vi "Pfeiffer-RVC300.get revision.vi"(0 "i ref in":refnum<vi>, 3 "ms timeout (10000)":i32=10000, 5 "error in (no error)":errorcluster) -> (14 "i ref out":refnum<vi>, 16 "revision":string, 17 "timed out":bool, 19 "error out":errorcluster)   [LabVIEW 2014, in "Pfeiffer-RVC300.lvlib"]
doc: "Queries the revision number from the device and creates the deviceID.\n\nLicense Agreement for this software:\n\nCopyright (C)\nMax-Planck-Institut für Kernphysik\nSaupfercheckweg 1\n69117 Heidelberg\nGermany\n\nContact: christopher.borgmann@mpi-hd.mpg.de\n\nThis program is free software: you can redistribute it and/or modify \nit under the terms of the GNU General Public License as published by\nthe Free Software Foundation, either version 3 of the License, or\n(at your option) any later version.\n\nThis program is distributed in the hope that it will be useful,\nbut WITHOUT ANY WARRANTY; without even the implied warranty of\nMERCHANTABILITY or FITNESS FOR A PARTICULAR PURPOSE. See the\nGNU General Public License for more details.\n\nYou should have received a copy of the GNU General Public License\nalong with this program. If not, see <http://www.gnu.org/licenses/>.\n\nMax-Planck-Institut für Kernphysik\nSaupfercheckweg 1, 69117 Heidelberg, Germany\nFor all questions and ideas contact: christopher.borgmann@mpi-hd.mpg.de\nLast update: 08.07.2010"
uses:
  Pfeiffer-RVC300.lvlib
  CSCore/CSApplicationBaseClasses/DeviceBase/DeviceBase.lvlib
  CSlibraries-extern/DimLVEvent/NodeMon-LV/LVNodeInfo/LVNodeInfo.lvlib
  CSlibraries/UtilityLib/UtilityLib.lvlib
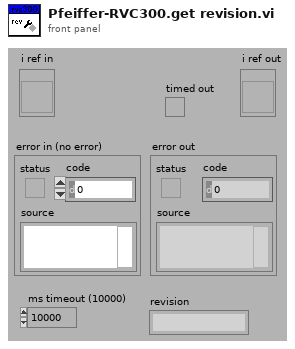
[diagram p1: front panel]
types:
  T1 = typedef "Pfeiffer-RVC300.lvlib/Pfeiffer-RVC300.i attribute.ctl" = cluster{"interfaceInitialized":bool, "VISAResource":refnum<visa-resource-name>, "WaitingTime":u32, "nomValues":T2, "actValues":T2}
  T2 = typedef "Pfeiffer-RVC300.lvlib/Pfeiffer-RVC300.parameters.ctl" = cluster{"regulationMode":T3, "valveType":string, "sensorType":string, "valveState":string, "flow":dbl, "pressure":dbl, "serviceIDs":cluster{"regulationModeID":i32, "valveTypeID":i32, "sensorTypeID":i32, "valveStateID":i32, "flowID":i32, "pressureID":i32}}
  T3 = typedef "Pfeiffer-RVC300.lvlib/Pfeiffer-RVC300.regulation mode.ctl" = enum16{"unknown", "Pressure", "Flow", "Wait"}
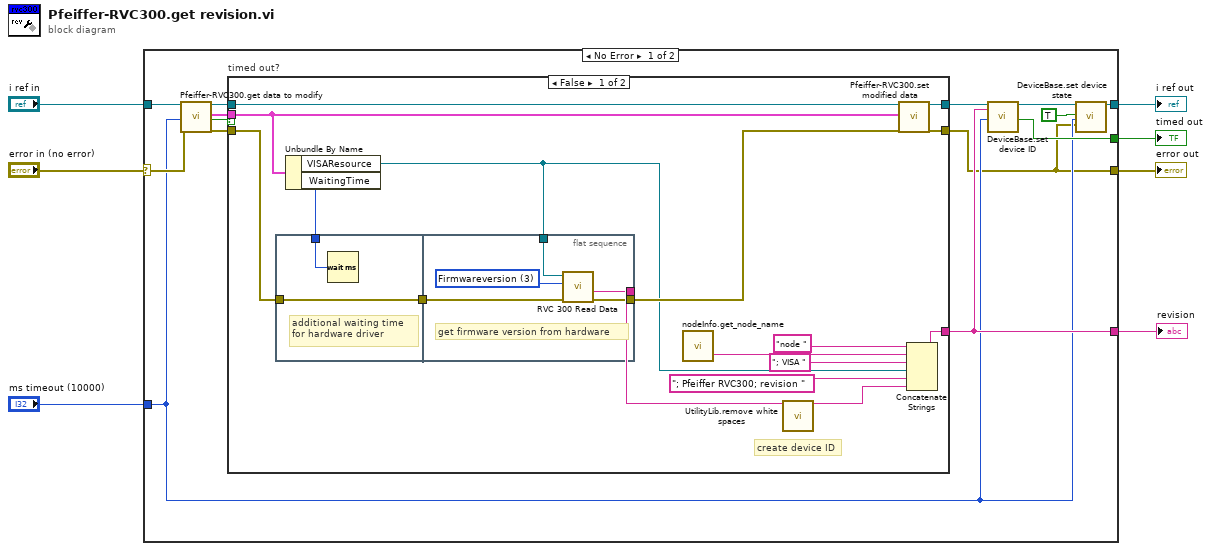
[diagram p0: block diagram]
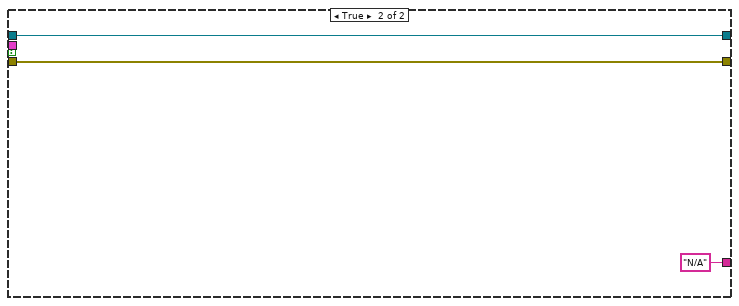
[diagram p2: hidden frame]
diagram:
  n1 = case shown="No Error" "error in (no error)" {
    selector: "error in (no error)" -> [w20 w48]
    tunnel: "i ref in" -> [w21 w49]
    tunnel: "ms timeout (10000)" -> [w10 _]
    tunnel: [w15 w49] -> w5
    tunnel: [w8 w48] -> w4
    tunnel: [w13 _] -> w2
    tunnel: [w17 _] -> w1
    frame No Error {
      n2 = call "Pfeiffer-RVC300.get data to modify.vi"("i ref in"=w21, "ms timeout (10000)"=w10, "error in (no error)"=w20) -> ("i ref out"=w11:refnum<vi>, "i attribute"=w18:T1, "timed out"=w12:bool, "error out"=w19:errorcluster)  [unwired: 13 in]
      n3 = case "timed out?" shown="False" w12 {
        tunnel: w19 -> [w27 w46]
        tunnel: w18 -> [w29 _]
        tunnel: [w34 "N/A"] -> w13
        tunnel: [w32 w46] -> w8
        tunnel: w11 -> [w33 w47]
        tunnel: [w31 w47] -> w9
        frame False {
          # "create device ID"
          n4 = flat-sequence {
            tunnel: w27 -> [w39]
            tunnel: [w39] -> w26
            tunnel: w23 -> [w38]
            tunnel: [w44] -> w25
            tunnel: [w42] -> w28
            tunnel: w26 -> [w41]
            tunnel: w22 -> [w40]
            frame #0 {
              # "additional waiting time \nfor hardware driver"
              n5 = Wait (ms)(milliseconds to wait=w38) -> ()  [unwired: 1 out]
            }
            frame #1 {
              w43 = u16 3 items=["Mode", "Pressure", "Unit", "Firmwareversion", "Keyboard lock", "Pressure Setpoint", "Sensor Type", "Valve Type"] ("RVC 300 Read")
              # "get firmware version from hardware"
              n6 = call "RVC 300 Read Data.vi"("error in"=w41, "RVC 300 Read"=w43, "Resource Name"=w40) -> ("error out"=w42:errorcluster, "Response Data out"=w44:string)  [unwired: 5 in, 2 out]
            }
          }
          n7 = Unbundle By Name(w29) -> ("VISAResource"=w22:refnum<visa-resource-name>, "WaitingTime"=w23:u32)
          n8 = call "nodeInfo.get_node_name.vi"() -> ("nodeName"=w36:string)  [unwired: 18 in, 1 out]
          n9 = call "UtilityLib.remove white spaces.vi"("string with blanks"=w25) -> ("string without white spaces"=w24:string)  [unwired: 14 in, 4 out]
          n10 = call "Pfeiffer-RVC300.set modified data.vi"("i ref in"=w33, "i attribute"=w29, "error in (no error)"=w28) -> ("i ref out"=w31:refnum<vi>, "error out"=w32:errorcluster)  [unwired: 15 in]
          n11 = Concatenate Strings("node " ("string"), w36, "; VISA " ("string"), w22, "; Pfeiffer RVC300; revision " ("string"), w24) -> (w34:string)
        }
        frame True {
        }
      }
      n12 = call "DeviceBase.set device ID.vi"("i ref in"=w9, "deviceID"=w13, "ms timeout (10000)"=w10) -> ("i ref out"=w16:refnum<vi>, "timed out"=w17:bool)  [unwired: 14 in, 1 out]
      n13 = call "DeviceBase.set device state.vi"("i ref in"=w16, "implicit"=TRUE, "ms timeout (10000)"=w10, "device error"=w8) -> ("i ref out"=w15:refnum<vi>)  [unwired: 13 in, 2 out]
    }
    frame Error {
    }
  }
  "error out" <- w4
  "i ref out" <- w5
  "timed out" <- w1
  "revision" <- w2
